vi "Excit_Extract_One_Wfm_From_Table.vi"(6 "Excitation Number":i32, 8 "error in (no error)":errorcluster, 9 "Sampling Frequency":dbl, 10 "Waveforms Table":string[](array[string])) -> (0 "error out":errorcluster caption="sortie d'erreur", 1 "Waveform Name":string, 2 "Excitation FFT":cluster{dbl[], "Power Spectrum (V^2 rms)":dbl[]}(graph), 3 "Excitation Signal":T2(graph), 4 "FIFO used":i32, 5 "Signal Excitation":dbl[](array[numeric]))   [LabVIEW 2020]
uses:
  controls/EXCIT_Form_Selector.ctl
  controls/EXCIT_Waveform_Inputs.ctl
panel:
  in  "Excit Form":T1=enum."Chirp"
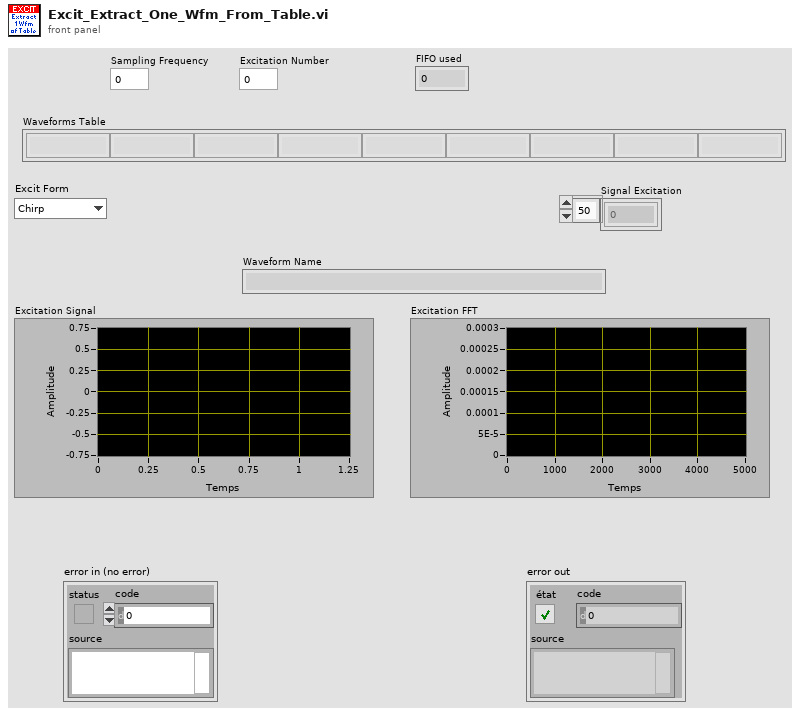
[diagram p1: front panel]
types:
  T1 = typedef "EXCIT_Form_Selector.ctl" = enum16{"Swift", "TwoSwift", "Chirp", "Sinus", "Ramp"}
  T2 = cluster{"X Time":dbl[], "Signal Excitation":dbl[]}
  T3 = typedef "EXCIT_Waveform_Inputs.ctl" = cluster{"Excit Form":T1, "Swift Factor":dbl, "Chirp Apodisation":dbl, "Duration":dbl, "Intensity":dbl, "Start Frequency":dbl, "End Frequency":dbl, "Intensity 2":dbl, "Start Frequency 2":dbl, "End Frequency 2":dbl, "Sampling Frequency":dbl}
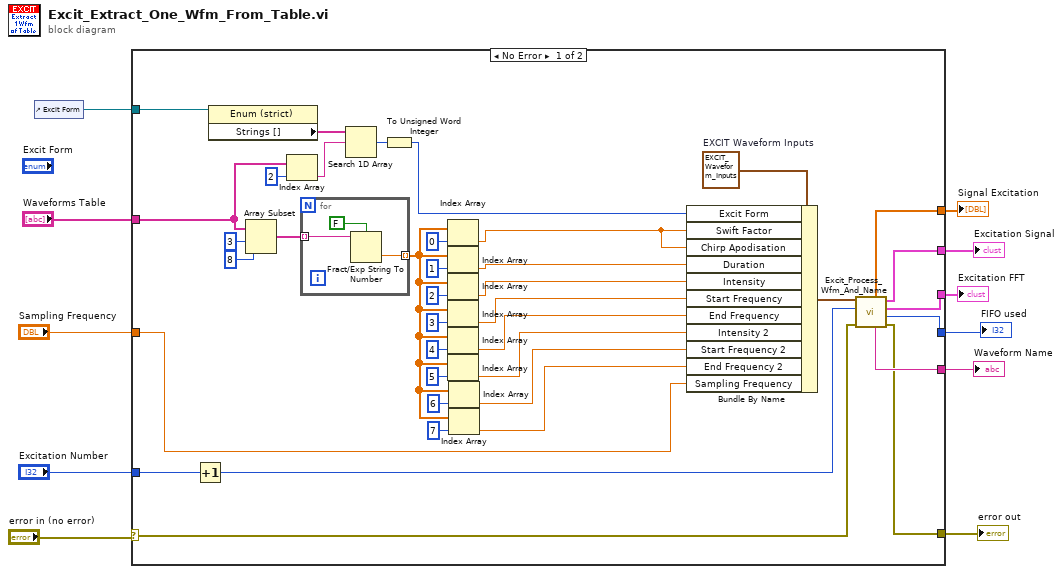
[diagram p0: block diagram]
diagram:
  n1 = control-ref of="Excit Form"() -> (w2:refnum<vi>)
  n2 = case shown="No Error" "error in (no error)" {
    selector: "error in (no error)" -> [w18 w54]
    tunnel: [w49 _] -> w11
    tunnel: [w48 _] -> w10
    tunnel: "Excitation Number" -> [w46 _]
    tunnel: "Sampling Frequency" -> [w44 _]
    tunnel: "Waveforms Table" -> [w29 _]
    tunnel: [w17 w54] -> w5
    tunnel: [w16 _] -> w4
    tunnel: [w15 _] -> w3
    tunnel: w2 -> [w13 _]
    tunnel: [w12 _] -> w1
    frame No Error {
      w32 = T3 {"Excit Form"=enum."Swift", "Swift Factor"=0.5, "Chirp Apodisation"=3.5, "Duration"=800.0, "Intensity"=100.0, "Start Frequency"=250.0, "End Frequency"=1000.0, "Intensity 2"=100.0, "Start Frequency 2"=250.0, "End Frequency 2"=350.0, "Sampling Frequency"=10.0}  # EXCIT Waveform Inputs
      n3 = Increment(x=w46) -> (x+1=w47:i32)
      n4 = property on="Nœud de propriété" class="Enum (strict)"(reference=w13) -> ("Strings []"=w50:string[])  [unwired: 1 in, 2 out]
      n5 = Array Subset(array=w29, index=3 ("indice"), length=8 ("longueur")) -> (w21:string[])
      n6 = Index Array(array=w29, index=2 ("indice")) -> (element=w27:string)
      n7 = for {
        tunnel: w21 -> [w53] mode=indexing
        tunnel: [w51] -> w31 mode=indexing
        n8 = Fract/Exp String To Number(use system decimal point (T)=FALSE ("utiliser le séparateur décimal du système (V)"), string=w53) -> (number=w51:dbl)  [unwired: 2 in, 1 out]
      }
      n9 = Search 1D Array(1D array=w50, element=w27) -> (index of element=w28:i32)  [unwired: 1 in]
      n10 = To Unsigned Word Integer(number=w28) -> (unsigned 16bit integer=w14:u16)
      n11 = Index Array(array=w31, index=0 ("indice")) -> (element=w33:dbl)
      n12 = Index Array(array=w31, index=1 ("indice")) -> (element=w34:dbl)
      n13 = Index Array(array=w31, index=2 ("indice")) -> (element=w35:dbl)
      n14 = Index Array(array=w31, index=3 ("indice")) -> (element=w36:dbl)
      n15 = Index Array(array=w31, index=4 ("indice")) -> (element=w37:dbl)
      n16 = Index Array(array=w31, index=5 ("indice")) -> (element=w41:dbl)
      n17 = Index Array(array=w31, index=6 ("indice")) -> (element=w42:dbl)
      n18 = Index Array(array=w31, index=7 ("indice")) -> (element=w43:dbl)
      n19 = Bundle By Name(cluster=w32, "Excit Form"=w14, "Swift Factor"=w33, "Chirp Apodisation"=w33, "Duration"=w34, "Intensity"=w35, "Start Frequency"=w36, "End Frequency"=w37, "Intensity 2"=w41, "Start Frequency 2"=w42, "End Frequency 2"=w43, "Sampling Frequency"=w44) -> (w45:T3)
      n20 = call "Excit_Process_Wfm_And_Name.vi"("error in (no error)"=w18, "Excit Number"=w47, "EXCIT Waveform Inputs"=w45) -> ("error out"=w17:errorcluster, "FIFO used"=w12:i32, "Excitation FFT"=w15:cluster{dbl[], "Power Spectrum (V^2 rms)":dbl[]}, "Excitation Signal"=w49:T2, "Waveform Name"=w48:string, "Signal Excitation"=w16:dbl[])  [unwired: 3 in]
    }
    frame Error {
    }
  }
  "Excitation Signal" <- w11
  "Waveform Name" <- w10
  "error out" <- w5
  "Signal Excitation" <- w4
  "Excitation FFT" <- w3
  "FIFO used" <- w1
